vi "PBPCIcard_close.vi"(0 "error in":errorcluster) -> (1 "Error?":bool, 2 "error out":errorcluster)   [LabVIEW 2013]
doc: "This VI puts the PulseBlaster board in non-programmable mode. 'PBPCIcard_init' puts the PB card in programmable mode to begin with. It is not necessary to switch the card between modes very often, if at all. I think it would only be necessary for trouble shooting purposes."
uses:
  WINDOWS/system32/PBD03PC.dll
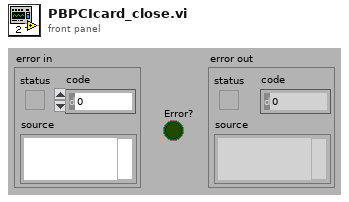
[diagram p1: front panel]
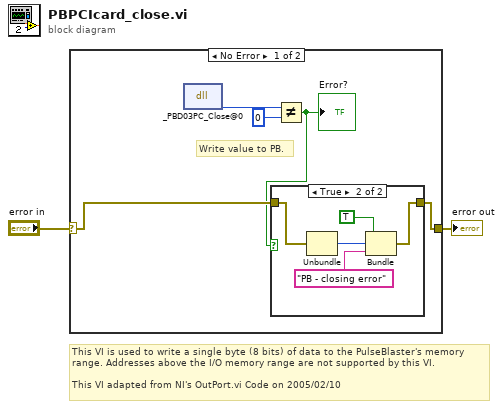
[diagram p0: block diagram]
diagram:
  # "This VI is used to write a single byte (8 bits) of data to the PulseBlaster's memory range. Addresses above the I/O memory range are not supported by this VI.\n\nThis VI adapted from NI's OutPort.vi Code on 2005/02/10"
  n1 = case shown="No Error" "error in" {
    selector: "error in" -> [w5 w14]
    tunnel: [w4 w14] -> w2
    frame No Error {
      # "Write value to PB."
      n2 = dll-call lib="C:/WINDOWS/system32/PBD03PC.dll" fn="_PBD03PC_Close@0" label="Call Library Function Node"() -> (w6:i8)  [unwired: 3 in, 2 out]
      n3 = Not Equal?(x=w6, y=0) -> (x != y?=w3:bool)
      "Error?" <- w3
      n4 = case shown="True" w3 {
        tunnel: w5 -> [w8 w13]
        tunnel: [w8 w12] -> w4
        frame False {
        }
        frame True {
          n5 = Unbundle(w13) -> ("code"=w10:i32)  [unwired: 2 out]
          n6 = Bundle(TRUE, "code"=w10, "PB - closing error") -> (w12:cluster{bool, "code":i32, string})  [unwired: 1 in]
        }
      }
    }
    frame Error {
      # "Error was passed in.\nDo nothing."
    }
  }
  "error out" <- w2
